vi "SRDG535.PC Set Trigger.vi"(0 "i ref in":refnum<vi>, 2 "Trigger Settings":T1={"trigger"=0, "Impedance"=FALSE, "Slope"=FALSE, "burst count"=2, "external level (V)"=0.0, "Internal/Burst Rate (Hz)"=0.001, "Burst Period"=4} {"Burst Period" min=4 max=32766; "Internal/Burst Rate (Hz)" min=0.001 max=1000000.0 format="%.3f"; "external level (V)" min=-2.56 max=2.56 format="%.2f"; "burst count" min=2 max=32766; "trigger" scale=0.0..4.0}, 5 "error IO":errorcluster) -> (14 "i ref out":refnum<vi>, 19 "error out":errorcluster)   [LabVIEW 2014, in "SRDG535.lvlib"]
doc: "This VI communicates with the hardware, sets own attributes and GUI elements."
uses:
  SRDG535.lvlib
  SRDG535.Trigger.ctl
  CSPhelix/PH_Common/PH_Common.lvlib
  non_GPL/instr.lib/srdg535/Stanford Research DG535 - Driver np.lvlib
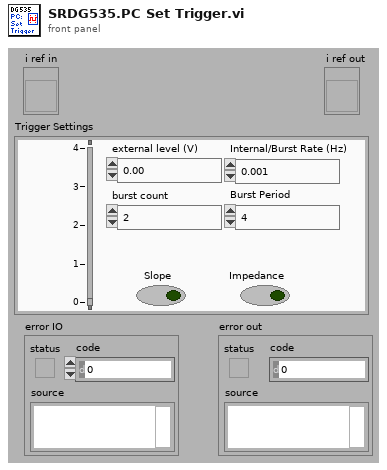
[diagram p1: front panel]
types:
  T1 = typedef "SRDG535.lvlib/SRDG535.Trigger.ctl" = cluster{"trigger":u32, "Impedance":bool, "Slope":bool, "burst count":i32, "external level (V)":sgl, "Internal/Burst Rate (Hz)":dbl, "Burst Period":i32}
  T2 = typedef "SRDG535.lvlib/SRDG535.i attribute.ctl" = cluster{"GPIB address":string, "Device error":errorcluster, "GUI Refs":cluster{"Delete":refnum<vi>, "Device Error":refnum<vi>, "Information":refnum<vi>, "Output":refnum<vi>, "Delay":refnum<vi>, "Trigger":refnum<vi>}, "Output Settings":T3, "Service ID Rate":i32, "Service IDs Channelinfo":i32[], "Delay Settings":T5, "Trigger Settings":T1}
  T3 = typedef "SRDG535.lvlib/SRDG535.Output.ctl" = cluster{"CH T0":T4, "CH A":T4, "CH B":T4, "CH AB":T4, "CH C":T4, "CH D":T4, "CH CD":T4}
  T4 = typedef "SRDG535.lvlib/SRDG535.Channel Output.ctl" = cluster{"Inversion":bool, "Amplitude (V)":dbl, "Offset (V)":dbl, "Mode":i32, "Load":bool}
  T5 = typedef "SRDG535.lvlib/SRDG535.Delay.ctl" = cluster{"CH A":cluster{"rel to":u32, "Delay (s)":dbl}, "CH B":cluster{"rel to":u32, "Delay (s)":dbl}, "CH C":cluster{"rel to":u32, "Delay (s)":dbl}, "CH D":cluster{"rel to":u32, "Delay (s)":dbl}}
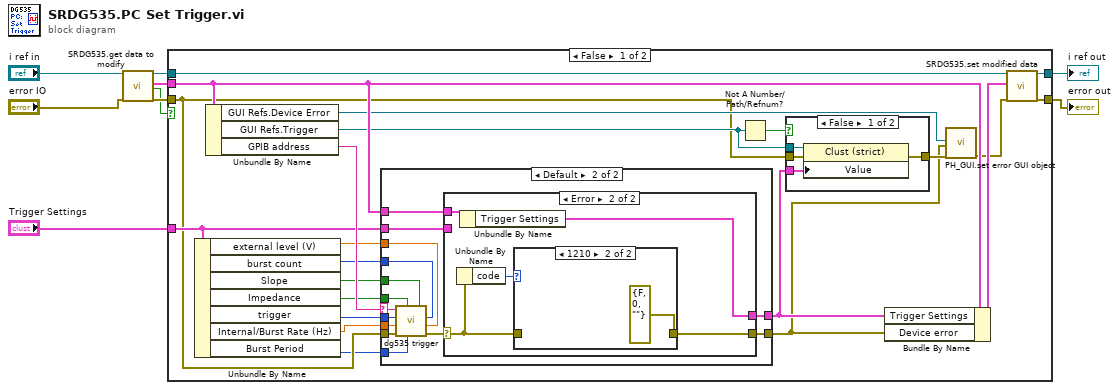
[diagram p0: block diagram]
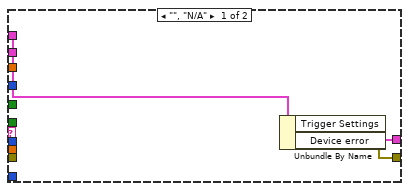
[diagram p3: hidden frame]
diagram:
  n1 = call "SRDG535.get data to modify.vi"("i ref in"="i ref in", "error in (no error)"="error IO") -> ("i ref out"=w5:refnum<vi>, "i attribute"=w9:T2, "timed out"=w2:bool, "error out"=w7:errorcluster)  [unwired: 14 in]
  n2 = case shown="False" w2 {
    tunnel: w9 -> [w31 _]
    tunnel: [w29 w63] -> w8
    tunnel: w7 -> [w19 w63]
    tunnel: [w28 w64] -> w6
    tunnel: w5 -> [w27 w64]
    tunnel: "Trigger Settings" -> [w20 _]
    frame False {
      n3 = Unbundle By Name(w20) -> ("external level (V)"=w18:sgl, "burst count"=w17:i32, "Slope"=w16:bool, "Impedance"=w15:bool, "trigger"=w14:u32, "Internal/Burst Rate (Hz)"=w13:dbl, "Burst Period"=w12:i32)
      n4 = Unbundle By Name(w31) -> ("GUI Refs.Device Error"=w26:refnum<vi>, "GUI Refs.Trigger"=w22:refnum<vi>, "GPIB address"=w25:string)
      n5 = case shown="Default" w25 {
        selector: w25 -> [_ w49]
        tunnel: w19 -> [_ w51]
        tunnel: [w38 w53] -> w10
        tunnel: w31 -> [w39 w52]
        tunnel: [w37 w48] -> w11
        tunnel: w20 -> [_ w47]
        tunnel: w18 -> [_ w46]
        tunnel: w17 -> [_ w45]
        tunnel: w16 -> [_ w44]
        tunnel: w15 -> [_ w43]
        tunnel: w14 -> [_ w42]
        tunnel: w13 -> [_ w41]
        tunnel: w12 -> [_ w40]
        frame "", "N/A" {
          n6 = Unbundle By Name(w39) -> ("Trigger Settings"=w37:T1, "Device error"=w38:errorcluster)
        }
        frame Default {
          n7 = call "dg535 trigger.vi"("external trigger level"=w46, "burst count"=w45, "trigger slope"=w44, "burst period"=w40, "input impedance"=w43, "error in"=w51, "internal/burst trigger rate"=w41, "trigger"=w42, "GPIB address"=w49) -> ("error out"=w50:errorcluster)
          n8 = case shown="Error" w50 {
            selector: w50 -> [w55 w57]
            tunnel: [w55 w56] -> w53
            tunnel: w52 -> [_ w59]
            tunnel: [w54 w60] -> w48
            tunnel: w47 -> [w54 _]
            frame No Error {
            }
            frame Error {
              n9 = Unbundle By Name(w57) -> ("code"=w58:i32)
              n10 = Unbundle By Name(w59) -> ("Trigger Settings"=w60:T1)
              n11 = case shown="1210" w58 {
                tunnel: w57 -> [w61 _]
                tunnel: [w61 errorcluster {"status"=FALSE, "code"=0, "source"=""} ("error IO")] -> w56
                frame 0, Default {
                }
                frame 1210 {
                }
              }
            }
          }
        }
      }
      n12 = Not A Number/Path/Refnum?(number/path/refnum=w22) -> (NaN/Path/Refnum?=w21:bool)
      n13 = case shown="False" w21 {
        tunnel: [w35 w36] -> w23
        tunnel: w19 -> [w34 w36]
        tunnel: w22 -> [w33 _]
        tunnel: w11 -> [w32 _]
        frame False {
          n14 = property class="Clust (strict)"(reference=w33, error in=w34, "Value"=w32) -> (error out=w35:errorcluster)  [unwired: 1 out]
        }
        frame True {
        }
      }
      n15 = Bundle By Name(cluster=w31, "Trigger Settings"=w11, "Device error"=w10) -> (w30:T2)
      n16 = call "PH_GUI.set error GUI object.vi"("GUI Refs.Device Error"=w26, "error to set"=w10, "error in (no error)"=w23) -> ("error out"=w24:errorcluster)  [unwired: 16 in]
      n17 = call "SRDG535.set modified data.vi"("i ref in"=w27, "i attribute"=w30, "error in (no error)"=w24) -> ("i ref out"=w28:refnum<vi>, "error out"=w29:errorcluster)  [unwired: 15 in]
    }
    frame True {
    }
  }
  "error out" <- w8
  "i ref out" <- w6
